vi "Write Publisher Msg.vi"(8 "error in (no error)":errorcluster, 9 "Sender Enqueuer ID string":string, 10 "Message Priority(normal)":T1=enum."Normal", 11 "Publisher Msg in":refnum<class "Publisher Msg.lvclass">) -> (0 "error out":errorcluster, 3 "Publisher Msg out":refnum<class "Publisher Msg.lvclass">)   [LabVIEW 2020, in "Publisher.lvlib" / "Publisher Msg.lvclass"]
uses:
  Publisher Msg.lvclass
  PPL/HDH.Actor Framework.Core.Actor.lvlibp/1abvi3w/vi.lib/ActorFramework/Message Enqueuer/Message Priority.ctl
  Publisher Msg.lvclass/Publisher Msg.ctl
  PPL/HDH.Actor Framework.Core.Actor.lvlibp/1abvi3w/vi.lib/ActorFramework/Message Enqueuer/Message Enqueuer.lvclass
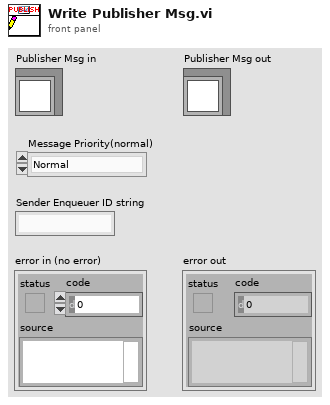
[diagram p1: front panel]
types:
  T1 = typedef "HDH.Actor Framework.Core.Actor.lvlibp/Message Enqueuer.lvclass/Message Priority.ctl" = enum16{"Low", "Normal", "High"}
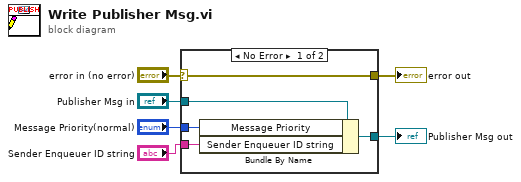
[diagram p0: block diagram]
diagram:
  n1 = case shown="No Error" "error in (no error)" {
    selector: "error in (no error)" -> [w11 w12]
    tunnel: [w11 w12] -> w5
    tunnel: [w9 w13] -> w3
    tunnel: "Publisher Msg in" -> [w10 w13]
    tunnel: "Sender Enqueuer ID string" -> [w8 _]
    tunnel: "Message Priority(normal)" -> [w7 _]
    frame No Error {
      n2 = Bundle By Name(cluster=w10, "Message Priority"=w7, "Sender Enqueuer ID string"=w8) -> (w9:refnum<class "Publisher Msg.lvclass">)
    }
    frame Error {
    }
  }
  "error out" <- w5
  "Publisher Msg out" <- w3
